vi "Ensenso_Receiver.vi"() -> ()   [LabVIEW 2015]
uses:
  <vilib>/Utility/tcp.llb/UDP Multicast Read-Write Open.vi
panel:
  in  "Tab Control":enum32{"Charts"}(tab)
  out "Translation":dbl[][](graph)
  out "Seq No":dbl
  out "x":dbl
  out "ROS Time":dbl
  in  "Stop":bool
  out "y":dbl
  out "z":dbl
  out "pitch":dbl
  out "Rotation":dbl[][](graph)
  out "error out":errorcluster
  out "yaw":dbl
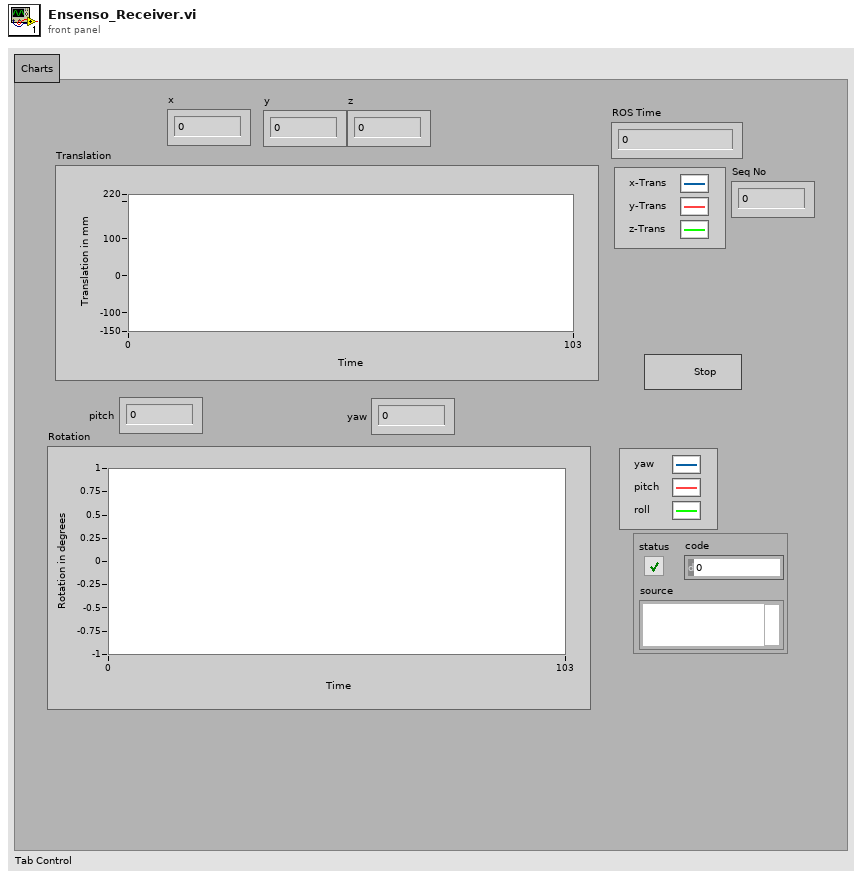
[diagram p1: front panel]
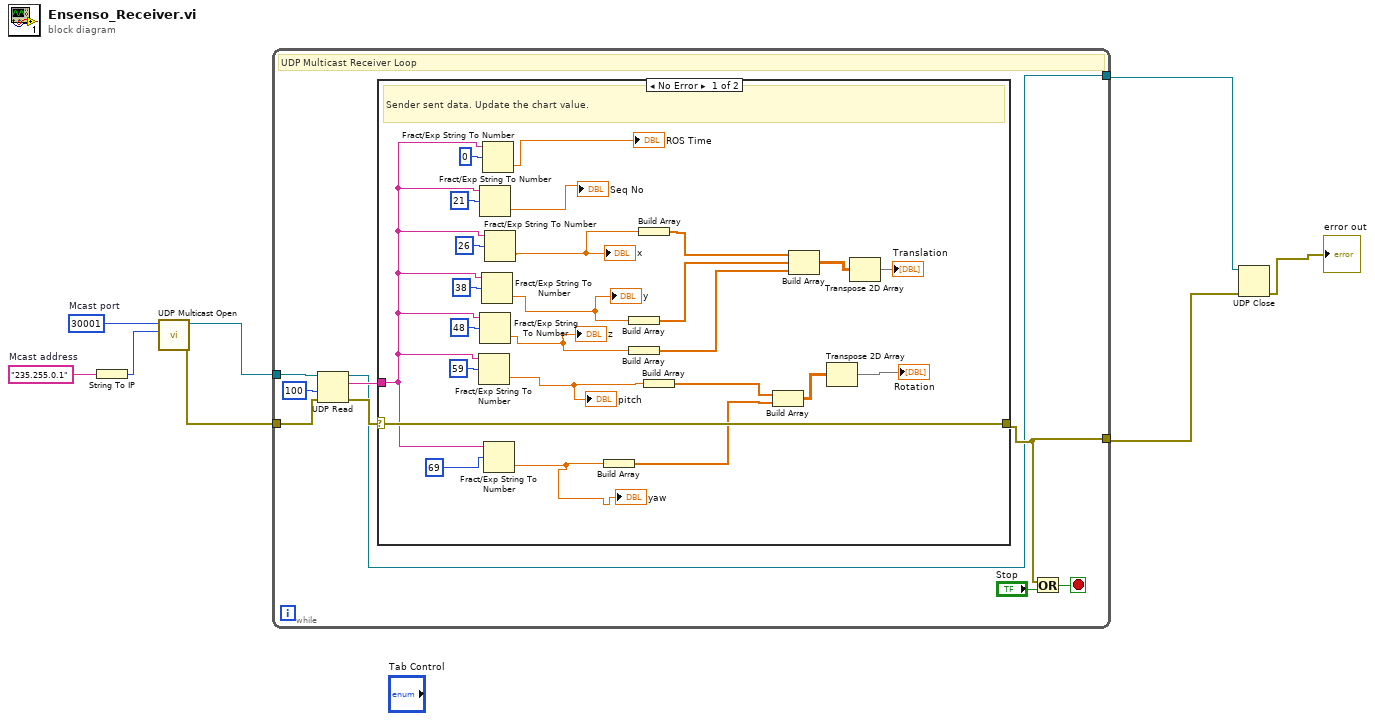
[diagram p0: block diagram]
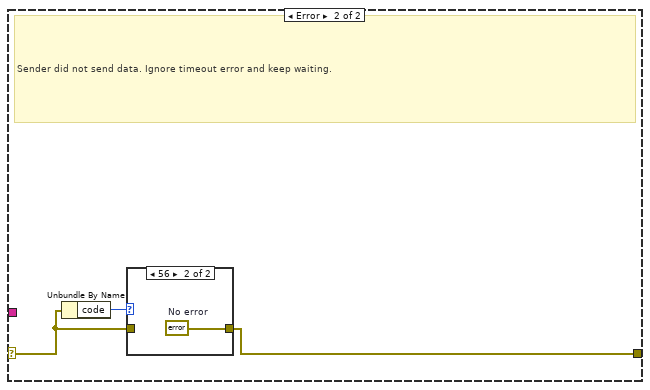
[diagram p2: hidden frame]
diagram:
  w3 = u16 30001  # Mcast port
  w7 = "235.255.0.1"  # Mcast address
  n1 = String To IP(1:w7) -> (0:w2:u32)
  n2 = call-poly <vilib>:"UDP Multicast Open.vi"("multicast addr"=w2, "port"=w3) -> ("error out"=w5:errorcluster, "connection ID"=w4:refnum<k16>)  [unwired: 7 in, 1 out]
  n3 = while {
    tunnel: w4 -> [w17]
    tunnel: [w9] -> w8
    tunnel: w5 -> [w14]
    tunnel: [w10] -> w6
    stop <- w15 stop-if-true
    # "UDP Multicast Receiver Loop"
    n4 = UDP Read(connection ID=w17, timeout ms (25000)=100, 8:w14) -> (data out=w12:string, error out=w11:errorcluster, 3:w9:refnum<k16>)  [unwired: 3 out]
    n5 = case shown="No Error" w11 {
      selector: w11 -> [w42 w44]
      tunnel: w12 -> [w25 _]
      tunnel: [w42 w43] -> w10
      frame No Error {
        # "Sender sent data. Update the chart value."
        n6 = Fract/Exp String To Number(string=w25, offset=59) -> (number=w30:dbl)  [unwired: 2 in, 1 out]
        "pitch" <- w30
        n7 = Fract/Exp String To Number(string=w25, offset=21) -> (number=→"Seq No":dbl)  [unwired: 2 in, 1 out]
        n8 = Fract/Exp String To Number(string=w25, offset=48) -> (number=w31:dbl)  [unwired: 2 in, 1 out]
        "z" <- w31
        n9 = Fract/Exp String To Number(string=w25, offset=38) -> (number=w32:dbl)  [unwired: 2 in, 1 out]
        "y" <- w32
        n10 = Fract/Exp String To Number(string=w25, offset=0) -> (number=→"ROS Time":dbl)  [unwired: 2 in, 1 out]
        n11 = Fract/Exp String To Number(string=w25, offset=69) -> (number=w18:dbl)  [unwired: 2 in, 1 out]
        "yaw" <- w18
        n12 = Fract/Exp String To Number(string=w25, offset=26) -> (number=w29:dbl)  [unwired: 2 in, 1 out]
        "x" <- w29
        n13 = Build Array(w18) -> (w20:dbl[])
        n14 = Build Array(w32) -> (w23:dbl[])
        n15 = Build Array(w31) -> (w22:dbl[])
        n16 = Build Array(w29) -> (w24:dbl[])
        n17 = Build Array(w30) -> (w21:dbl[])
        n18 = Build Array(w21, w20) -> (w34:dbl[][])
        n19 = Build Array(w24, w23, w22) -> (w19:dbl[][])
        n20 = Transpose 2D Array(2D array=w34) -> (transposed array=→"Rotation":dbl[][])
        n21 = Transpose 2D Array(2D array=w19) -> (transposed array=→"Translation":dbl[][])
      }
      frame Error {
        # "Sender did not send data. Ignore timeout error and keep waiting."
        n22 = Unbundle By Name(w44) -> ("code"=w45:i32)
        n23 = case shown="56" w45 {
          tunnel: w44 -> [w46 _]
          tunnel: [w46 w47] -> w43
          frame Default {
          }
          frame 56 {
            w47 = errorcluster {"status"=FALSE, "code"=0, "source"=""}  # No error
          }
        }
      }
    }
    n24 = Or(x=w10, y="Stop") -> (x .or. y?=w15:bool)
  }
  n25 = UDP Close(connection ID=w8, 8:w6) -> (error out=→"error out":errorcluster)  [unwired: 1 out]
